vi "Teleop Elevator Control.vi"(0 "Axes":T2, 1 "Button Cluster":T3, 2 "D-Pad":T1) -> ()   [LabVIEW 2017]
uses:
  Common Code/Gamepads/Button Cluster.ctl
  Common Code/Gamepads/Axes Cluster.ctl
  Common Code/Gamepads/D-Pad.ctl
  Common Code/Elevator Mode.ctl
  Common Code/Elevator State.ctl
  Robot Global Data.vi
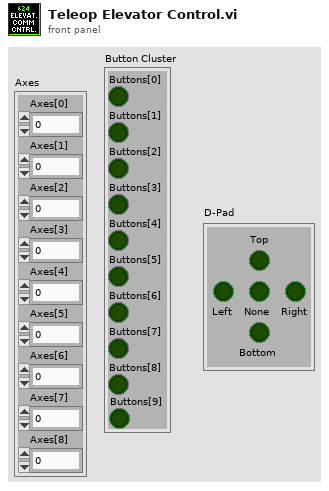
[diagram p1: front panel]
types:
  T1 = typedef "D-Pad.ctl" = cluster{"Top":bool, "Bottom":bool, "None":bool, "Right":bool, "Left":bool}
  T2 = typedef "Axes Cluster.ctl" = cluster{"Axes[0]":dbl, "Axes[1]":dbl, "Axes[2]":dbl, "Axes[3]":dbl, "Axes[4]":dbl, "Axes[5]":dbl, "Axes[6]":dbl, "Axes[7]":dbl, "Axes[8]":dbl}
  T3 = typedef "Button Cluster.ctl" = cluster{"Buttons[0]":bool, "Buttons[1]":bool, "Buttons[2]":bool, "Buttons[3]":bool, "Buttons[4]":bool, "Buttons[5]":bool, "Buttons[6]":bool, "Buttons[7]":bool, "Buttons[8]":bool, "Buttons[9]":bool}
  T4 = typedef "Elevator Mode.ctl" = enum16{"Manual", "Auto"}
  T5 = typedef "Dashboard Control Data.ctl" = cluster{"Drivetrain Settings Cluster":T6, "Intake Presets":T9, "Elevator Settings Cluster":T10}
  T6 = typedef "Drivetrain Settings Clustr.ctl" = cluster{"Gyro PID Gains":T7, "Drive PID Gains":T7, "Encoder Values":T8, "Drive Tolerance":dbl, "Gyro Tolerance":dbl, "Gyro Output":dbl, "Distance Output":dbl}
  T7 = typedef "PID Gains Cluster.ctl" = cluster{"Integral Time":dbl, "Proportional Gain":dbl, "Derivative Time":dbl}
  T8 = typedef "Encoder Values.ctl" = cluster{"Distance":dbl, "Speed":dbl, "Tick":dbl}
  T9 = typedef "Intake Presets.ctl" = cluster{"Idle Height":dbl, "Mid Height":dbl, "Low Height":dbl, "Outtake Power":dbl, "Intake Power":dbl, "Flick Power":dbl, "Unstuck":dbl, "Angle Tolerance":dbl, "Max Height":dbl, "Max Current":dbl, "Current Trip Time":dbl, "Reset Encoder?":bool, "Encoder Scale":dbl, "PID gains":cluster{"proportional gain (Kc)":dbl, "integral time (Ti, min)":dbl, "derivative time (Td, min)":dbl}, "output range":cluster{"output high":dbl, "output low":dbl}}
  T10 = typedef "Elevator Settings Cluster.ctl" = cluster{"Ground Height":dbl, "Switch Height":dbl, "Scale High Height ":dbl, "Scale Low Height":dbl, "Elevator PID Gains":T11, "High Output":dbl, "Low Output":dbl, "Elevator Tolerance":dbl, "Reset Encoders":bool}
  T11 = typedef "PID Gains.ctl" = cluster{"proportional gain (Kc)":dbl, "integral time (Ti, min)":dbl, "derivative time (Td, min)":dbl}
  T12 = typedef "Elevator Status Cluster.ctl" = cluster{"Finished":bool, "Output":dbl, "Elevator State":T13, "Elevator Mode":T4, "Encoder Height":dbl, "Overextending?":bool}
  T13 = typedef "Elevator State.ctl" = enum16{"Idle", "Ground", "Scale High", "Scale Low", "Switch"}
  T14 = typedef "WPI_SwitchDevRef.ctl" = cluster{"DevStatus":errorcluster, "DIO Channel":T15, "CntIndex":T16, "Normally Closed":bool}
  T15 = typedef "FPGA_DIOChannel.ctl" = enum8{"DIO 0", "DIO 1", "DIO 2", "DIO 3", "DIO 4", "DIO 5", "DIO 6", "DIO 7", "DIO 8", "DIO 9", "DIO MXP 0", "DIO MXP 1", "DIO MXP 2", "DIO MXP 3", "DIO MXP 4", "DIO MXP 5", "DIO MXP 6", "DIO MXP 7", "DIO MXP 8", "DIO MXP 9", "DIO MXP 10", "DIO MXP 11", "DIO MXP 12", "DIO MXP 13", "DIO MXP 14", "DIO MXP 15", "SPI Port CS1", "SPI Port CS2", "SPI Port CS3", "SPI Port MISO", "SPI Port MOSI", "Invalid"}
  T16 = typedef "FPGA_CounterCtrSystemIndex.ctl" = enum8{"Ctr 0", "Ctr 1", "Ctr 2", "Ctr 3", "Ctr 4", "Ctr 5", "Ctr 6", "Ctr 7", "Invalid"}
  T17 = typedef "Elevator Command Cluster.ctl" = cluster{"Elevator Mode":T4, "Elevator State":T13, "Manual Speed":dbl, "Reset Encoders":bool}
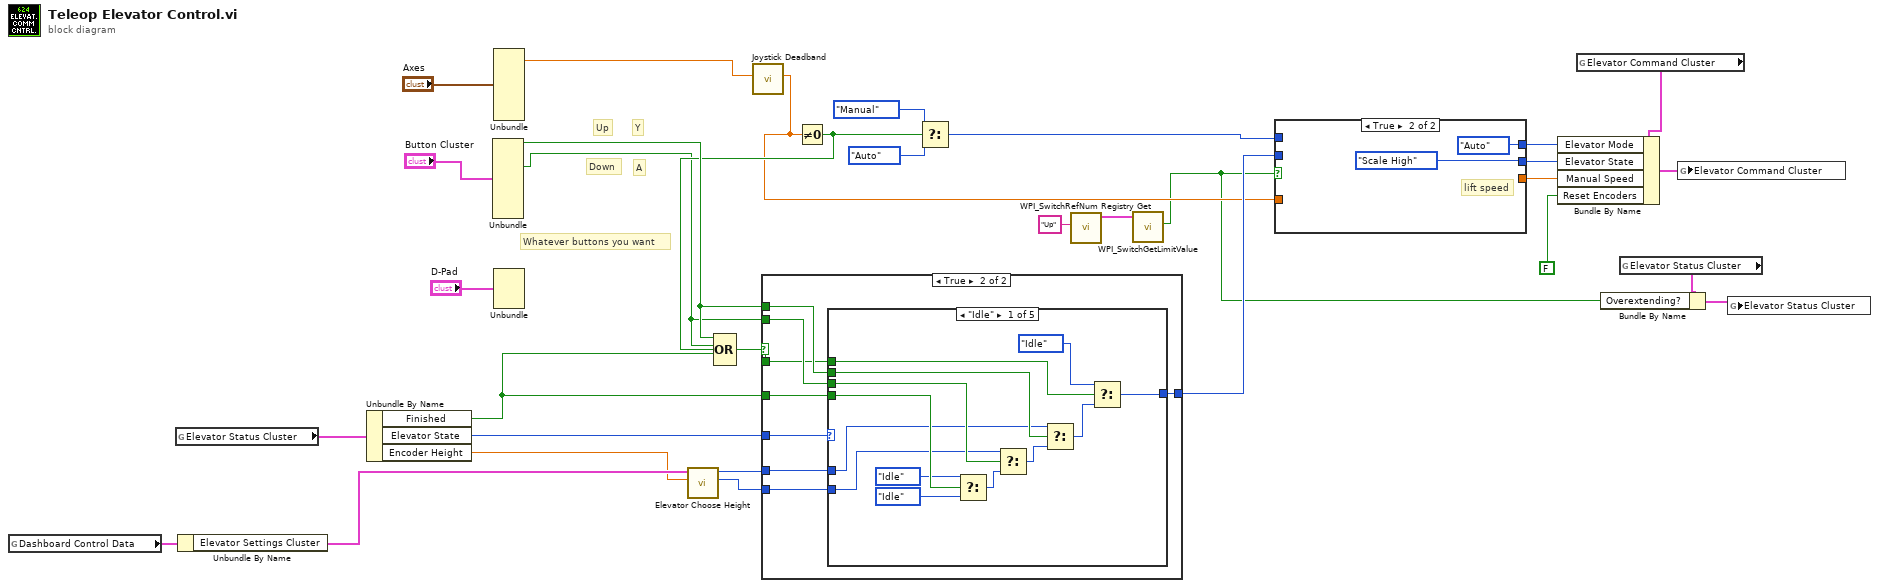
[diagram p0: block diagram]
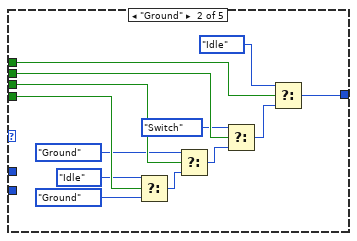
[diagram p4: hidden frame]
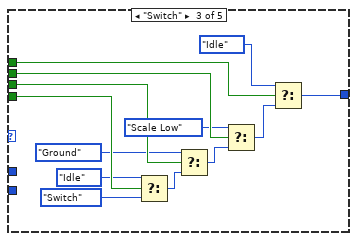
[diagram p5: hidden frame]
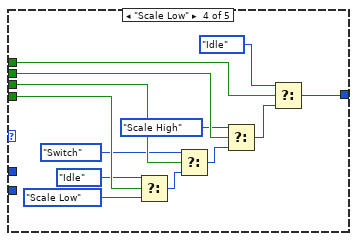
[diagram p6: hidden frame]
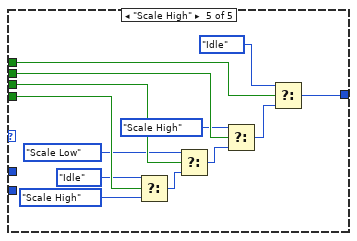
[diagram p7: hidden frame]
diagram:
  # "A"
  # "Y"
  # "Down"
  # "Up"
  # "Whatever buttons you want"
  n1 = global read "Robot Global Data.vi" "Dashboard Control Data"() -> (w20:T5)
  n2 = global read "Robot Global Data.vi" "Elevator Status Cluster"() -> (w27:T12)
  n3 = Unbundle By Name(w20) -> ("Elevator Settings Cluster"=w17:T10)
  n4 = Unbundle By Name(w27) -> ("Finished"=w23:bool, "Elevator State"=w24:T13, "Encoder Height"=w16:dbl)
  n5 = Unbundle("Button Cluster") -> ("Buttons[0]"=w25:bool, "Buttons[3]"=w15:bool)  [unwired: 8 out]
  n6 = Unbundle("Axes") -> ("Axes[1]"=w14:dbl)  [unwired: 8 out]
  n7 = Unbundle("D-Pad") -> ()  [unwired: 5 out]
  n8 = call "Elevator Choose Height.vi"("Encoder Height"=w16, "Elevator Settings Cluster"=w17) -> ("Down"=w18:T13, "Up"=w19:T13)  [unwired: 8 in]
  n9 = call "Joystick Deadband.vi"("In"=w14) -> ("Out"=w10:dbl)  [unwired: 10 in]
  n10 = Not Equal To 0?(x=w10) -> (x != 0?=w22:bool)
  n11 = Compound Arithmetic op=OR(w25, w15, w23, w22) -> (w26:bool)
  n12 = case shown="True" w26 {
    tunnel: w25 -> [_ w38]
    tunnel: w15 -> [_ w39]
    tunnel: [w33 w37] -> w11
    tunnel: w24 -> [w33 w41]
    tunnel: w23 -> [_ w40]
    tunnel: w22 -> [_ w36]
    tunnel: w19 -> [_ w35]
    tunnel: w18 -> [_ w34]
    frame False {
    }
    frame True {
      n13 = case shown="\"Idle\"" w41 {
        tunnel: w40 -> [w50 w63 w76 w89 w102]
        tunnel: w39 -> [w48 w61 w74 w87 w100]
        tunnel: w38 -> [w54 w67 w80 w93 w106]
        tunnel: [w46 w57 w70 w83 w96] -> w37
        tunnel: w36 -> [w45 w56 w69 w82 w95]
        tunnel: w35 -> [w43 _ _ _ _]
        tunnel: w34 -> [w42 _ _ _ _]
        frame "Idle" {
          n14 = Select(t=Elevator_State."Idle", s=w50, f=Elevator_State."Idle" ("Elevator State")) -> (s? t:f=w52:T13)
          n15 = Select(t=w42, s=w48, f=w52) -> (s? t:f=w53:T13)
          n16 = Select(t=w43, s=w54, f=w53) -> (s? t:f=w47:T13)
          n17 = Select(t=Elevator_State."Idle", s=w45, f=w47) -> (s? t:f=w46:T13)
        }
        frame "Ground" {
          n18 = Select(t=Elevator_State."Idle", s=w63, f=Elevator_State."Ground" ("Elevator State")) -> (s? t:f=w65:T13)
          n19 = Select(t=Elevator_State."Ground", s=w61, f=w65) -> (s? t:f=w66:T13)
          n20 = Select(t=Elevator_State."Switch", s=w67, f=w66) -> (s? t:f=w58:T13)
          n21 = Select(t=Elevator_State."Idle", s=w56, f=w58) -> (s? t:f=w57:T13)
        }
        frame "Switch" {
          n22 = Select(t=Elevator_State."Idle", s=w76, f=Elevator_State."Switch" ("Elevator State")) -> (s? t:f=w78:T13)
          n23 = Select(t=Elevator_State."Ground", s=w74, f=w78) -> (s? t:f=w79:T13)
          n24 = Select(t=Elevator_State."Scale Low", s=w80, f=w79) -> (s? t:f=w71:T13)
          n25 = Select(t=Elevator_State."Idle", s=w69, f=w71) -> (s? t:f=w70:T13)
        }
        frame "Scale Low" {
          n26 = Select(t=Elevator_State."Idle", s=w89, f=Elevator_State."Scale Low" ("Elevator State")) -> (s? t:f=w91:T13)
          n27 = Select(t=Elevator_State."Switch", s=w87, f=w91) -> (s? t:f=w92:T13)
          n28 = Select(t=Elevator_State."Scale High", s=w93, f=w92) -> (s? t:f=w84:T13)
          n29 = Select(t=Elevator_State."Idle", s=w82, f=w84) -> (s? t:f=w83:T13)
        }
        frame "Scale High" {
          n30 = Select(t=Elevator_State."Idle", s=w102, f=Elevator_State."Scale High" ("Elevator State")) -> (s? t:f=w104:T13)
          n31 = Select(t=Elevator_State."Scale Low", s=w100, f=w104) -> (s? t:f=w105:T13)
          n32 = Select(t=Elevator_State."Scale High", s=w106, f=w105) -> (s? t:f=w97:T13)
          n33 = Select(t=Elevator_State."Idle", s=w95, f=w97) -> (s? t:f=w96:T13)
        }
      }
    }
  }
  n34 = Select(t=Elevator_Mode."Manual", s=w22, f=Elevator_Mode."Auto" ("Elevator Mode")) -> (s? t:f=w7:T4)
  n35 = call <vilib>:"WPI_SwitchRefNum Registry Get.vi"("refnum name"="Up") -> ("SwitchDevRef"=w12:T14)  [unwired: 9 in, 1 out]
  n36 = call <vilib>:"WPI_SwitchGetLimitValue.vi"("SwitchDevRef"=w12) -> ("Switch Pressed"=w1:bool)  [unwired: 8 in, 2 out]
  n37 = case shown="True" w1 {
    tunnel: w11 -> [w109 _]
    tunnel: w10 -> [w108 _]
    tunnel: [w109 Elevator_State."Scale High" ("t")] -> w9
    tunnel: [w108 _] -> w8
    tunnel: w7 -> [w107 _]
    tunnel: [w107 Elevator_Mode."Auto" ("Elevator Mode")] -> w6
    frame False {
    }
    frame True {
      # "lift speed"
    }
  }
  n38 = global read "Robot Global Data.vi" "Elevator Command Cluster"() -> (w5:T17)
  n39 = Bundle By Name(cluster=w5, "Elevator Mode"=w6, "Elevator State"=w9, "Manual Speed"=w8, "Reset Encoders"=FALSE) -> (w4:T17)
  n40 = global read "Robot Global Data.vi" "Elevator Status Cluster"() -> (w3:T12)
  n41 = Bundle By Name(cluster=w3, "Overextending?"=w1) -> (w2:T12)
  n42 = global write "Robot Global Data.vi" "Elevator Command Cluster"(w4) -> ()
  n43 = global write "Robot Global Data.vi" "Elevator Status Cluster"(w2) -> ()
